vi "Autonomous Independent.vi"() -> ()   [LabVIEW 2011]
doc: "This VI is called when autonomous begins, and will automatically be terminated when autonomous ends. You can carry out timed or sensor driven robot movement independently without needing to return to the caller."
uses:
  <vilib>/addons/Kinect/Skeleton Vertex Index.ctl
  Robot Global Data.vi
  <vilib>/addons/control/pid/pid.llb/PID (DBL).vi
  <vilib>/addons/control/pid/NI_PID_pid.lvlib
panel:
  out "z 2":sgl
  out "y 2":sgl
  out "x 2":sgl
  out "z":sgl
  out "y":sgl
  out "x":sgl
  in  "PID gains":T1={"proportional gain (Kc)"=0.02, "integral time (Ti, min)"=0.0, "derivative time (Td, min)"=0.0}
  in  "setpoint":dbl=3000.0 format="%.2f"
  in  "PID gains 2":T1={"proportional gain (Kc)"=0.02, "integral time (Ti, min)"=0.0, "derivative time (Td, min)"=0.0}
  in  "setpoint 2":dbl=3300.0 format="%.2f"
  out "Left Distance 4":dbl
  out "Right Distance 4":dbl
  out "Right Distance 3":dbl
  out "Left Distance 3":dbl
  out "Left Distance 2":dbl
  out "Right Distance 2":dbl
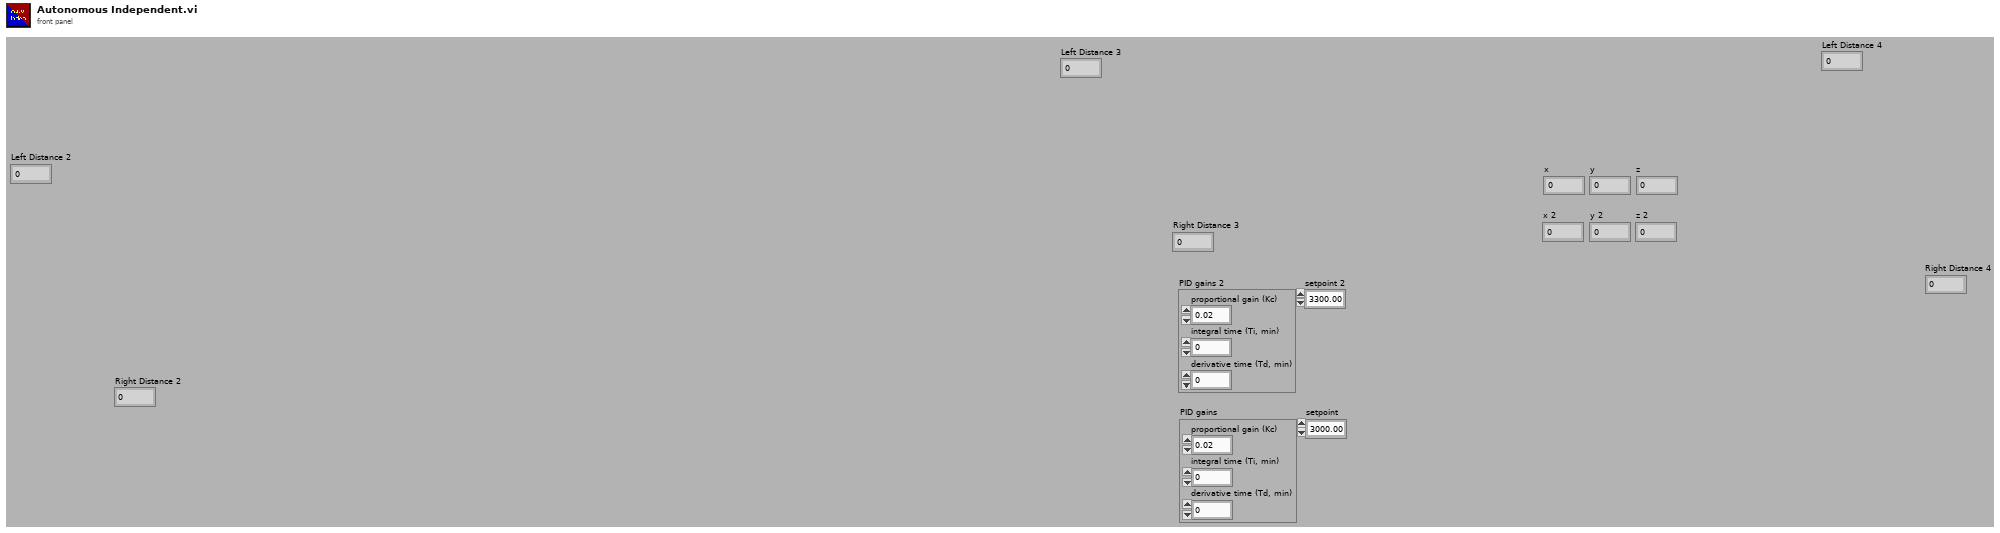
[diagram p1: front panel]
types:
  T1 = cluster{"proportional gain (Kc)":dbl, "integral time (Ti, min)":dbl, "derivative time (Td, min)":dbl}
  T2 = typedef "WPI_JoystickDevRef.ctl" = cluster{"Device":T3}
  T3 = typedef "WPI_JoystickDeviceEnum.ctl" = enum16{"USB 1", "USB 2", "USB 3", "USB 4", "Kinect 1", "Kinect 2"}
  T4 = cluster{"axis 1 (x)":dbl, "axis 2 (y)":dbl, "axis 3 (throttle)":dbl, "axis 4":dbl, "axis 5":dbl, "axis 6":dbl}
  T5 = typedef "Skeleton Vertex Index.ctl" = i32
  T6 = typedef "WPI_RobotDriveDevRef.ctl" = cluster{"DevStatus":errorcluster, "Motors[]":T7[], "Square Inputs":bool, "Max Output":dbl, "Isochronous":bool}
  T7 = typedef "WPI_MotorControlDeviceRef.ctl" = cluster{"DeviceStatus":errorcluster, "Type":enum16{"PWM", "CAN"}, "PWM":cluster{"Digital Module":T8, "PWM Channel":T9, "DeadBand":T10}, "CAN":cluster{"Device Number":u8, "Control Mode":T11, "Semaphore":T12, "Max Vout":dbl}, "Invert":bool, "TransformRef":T13, "InvTransformRef":T13}
  T8 = typedef "FPGA_TypedefDigitalModule.ctl" = enum16{"Digital Module 1", "Digital Module 2"}
  T9 = typedef "FPGA_DIOPWMChannel.ctl" = enum8{"PWM 1", "PWM 2", "PWM 3", "PWM 4", "PWM 5", "PWM 6", "PWM 7", "PWM 8", "PWM 9", "PWM 10", "Invalid"}
  T10 = typedef "WPI_PWMDeadband.ctl" = cluster{"Name":string, "maxPositivePwm":i32, "minPositivePwm":i32, "centerPwm":i32, "maxNegativePwm":i32, "minNegativePwm":i32, "angularRange":u16}
  T11 = typedef "WPI_CANJaguar_ControlMode.ctl" = enum8{"Percent VBus", "Current", "Speed", "Position", "Voltage"}
  T12 = typedef "Semaphore RefNum" = refnum<k1>
  T13 = typedef "WPI_PWMTransform_ConPane.ctl" = refnum<vi>
  T14 = typedef "WPI_EncoderDevRef.ctl" = cluster{"DevStatus":errorcluster, "EncoderIndex":T15, "CounterIndex":T16, "DistancePerCount":dbl, "Decoding Type":T17}
  T15 = typedef "FPGA_EncoderIdx.ctl" = enum8{"Enc 0", "Enc 1", "Enc 2", "Enc 3", "Invalid"}
  T16 = typedef "FPGA_CounterCtrSystemIndex.ctl" = enum8{"Ctr 0", "Ctr 1", "Ctr 2", "Ctr 3", "Ctr 4", "Ctr 5", "Ctr 6", "Ctr 7", "Invalid"}
  T17 = typedef "WPI_EncoderType.ctl" = enum16{"1x", "2x", "4x"}
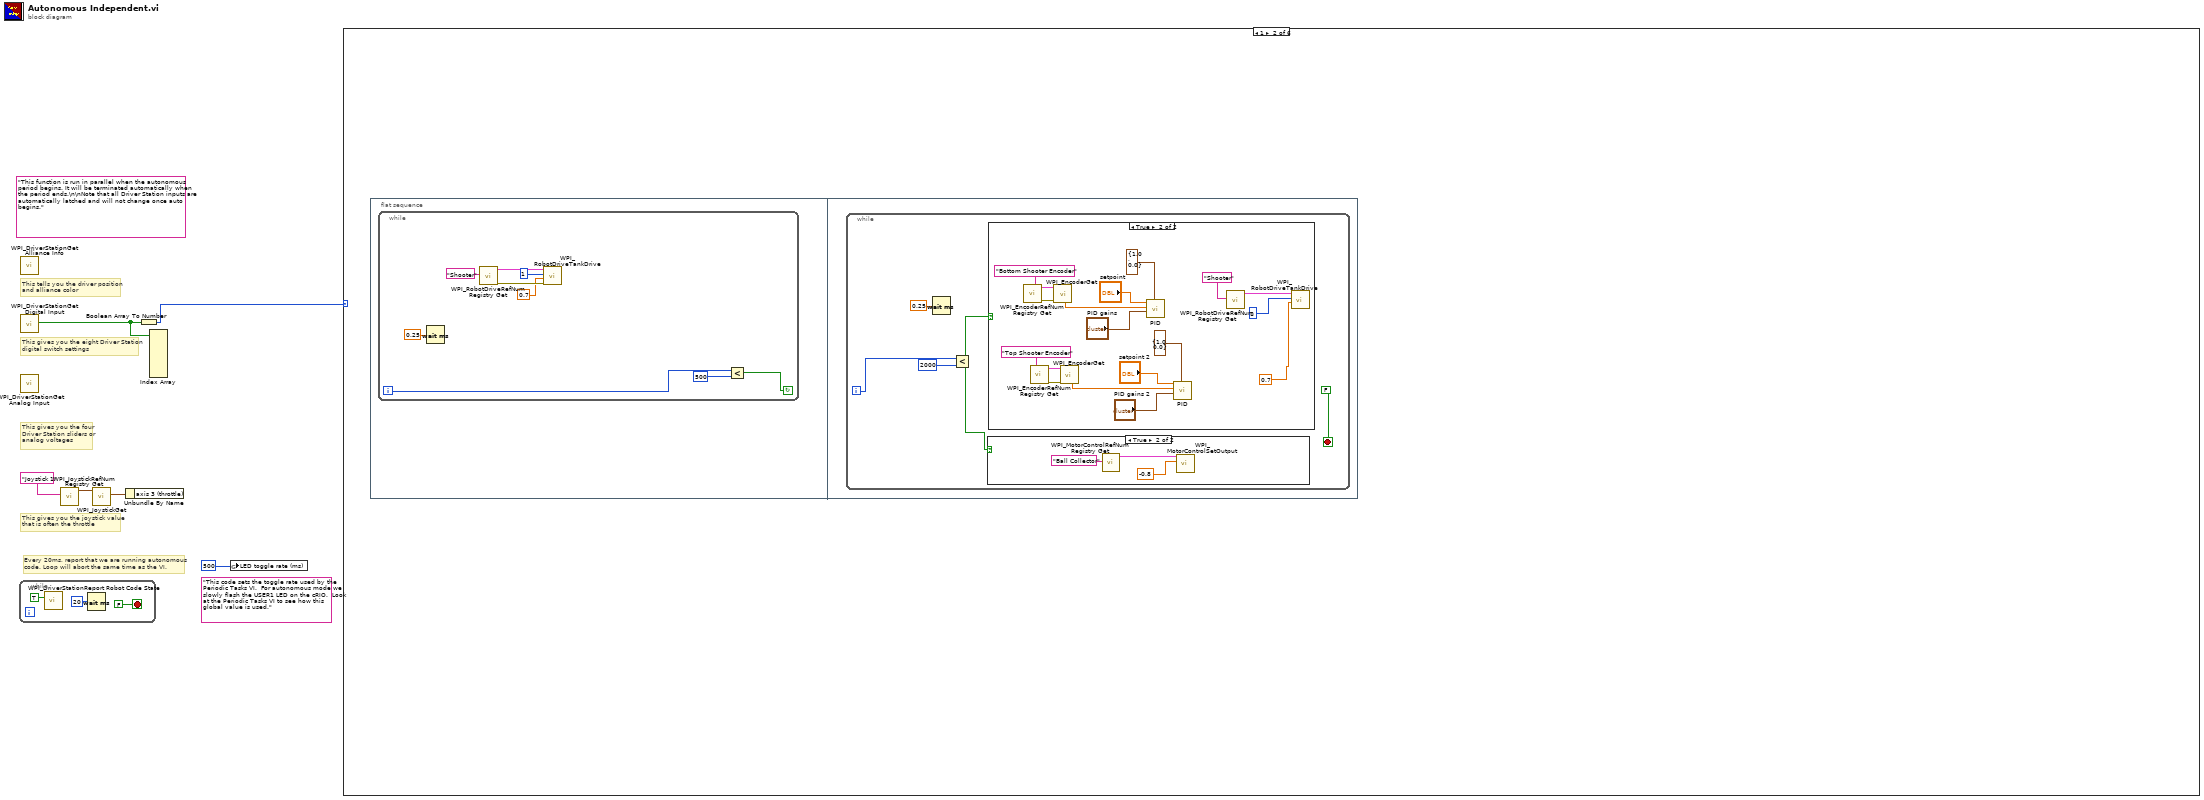
[diagram p0: block diagram]
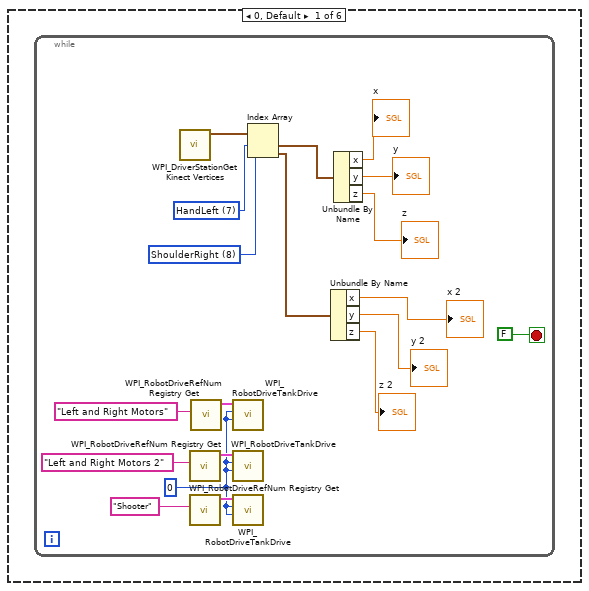
[diagram p2: hidden frame]
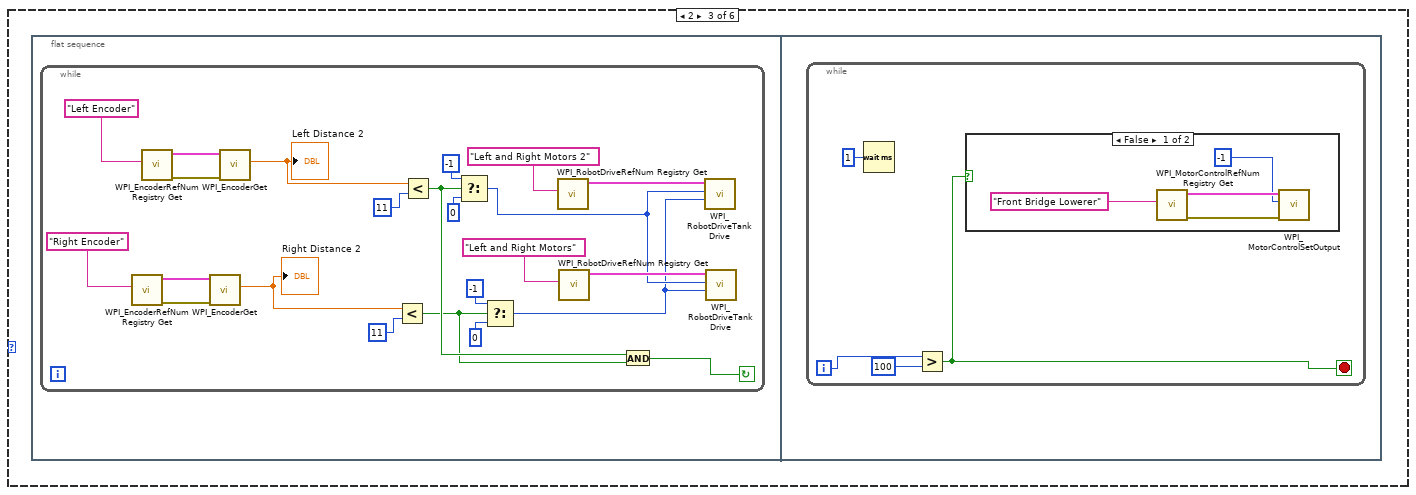
[diagram p5: hidden frame]
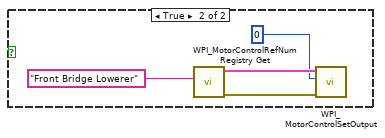
[diagram p6: hidden frame]
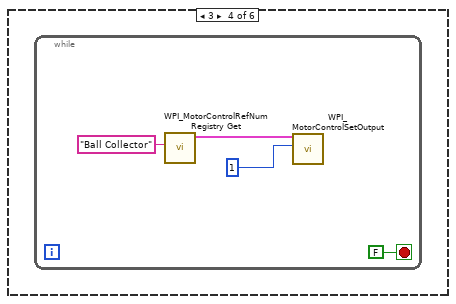
[diagram p7: hidden frame]
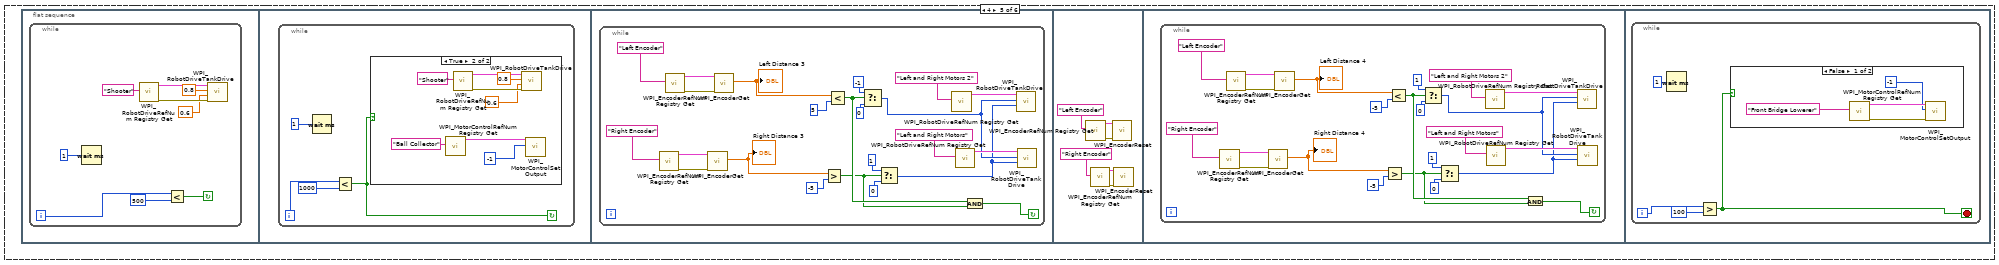
[diagram p8: hidden frame]
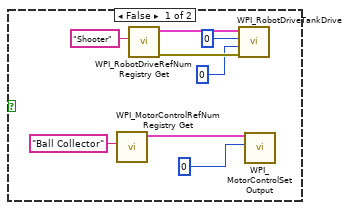
[diagram p9: hidden frame]
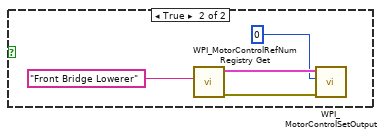
[diagram p10: hidden frame]
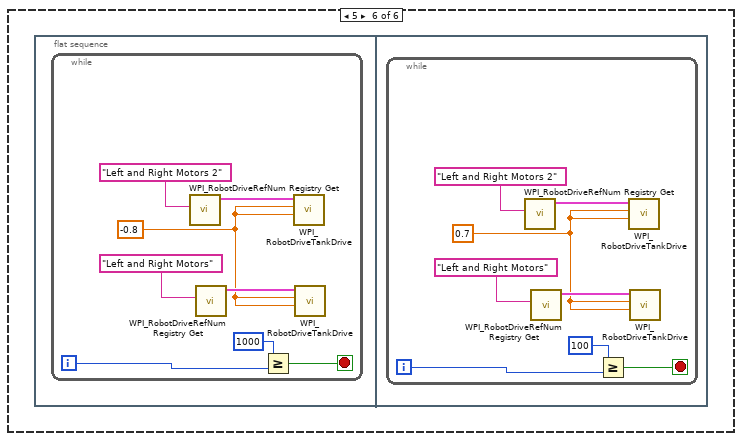
[diagram p11: hidden frame]
diagram:
  (unwired) "This code sets the toggle rate used by the Periodic Tasks VI.  For autonomous mode we slowly flash the USER1 LED on the cRIO.  Look at the Periodic Tasks VI to see how this global value is used."
  (unwired) "This function is run in parallel when the autonomous period begins. It will be terminated automatically when the period ends.\n\nNote that all Driver Station inputs are automatically latched and will not change once auto begins."
  # "Every 20ms, report that we are running autonomous\ncode. Loop will abort the same time as the VI."
  # "This gives you the joystick value\nthat is often the throttle"
  # "This tells you the driver position\nand alliance color"
  # "This gives you the eight Driver Station\ndigital switch settings"
  # "This gives you the four\nDriver Station sliders or\nanalog voltages"
  n1 = while {
    stop <- FALSE stop-if-true
    n2 = call <vilib>:"WPI_DriverStationReport Robot Code State.vi"("Autonomous"=TRUE) -> ()  [unwired: 10 in, 1 out]
    n3 = Wait (ms)(milliseconds to wait=u32 20) -> ()  [unwired: 1 out]
  }
  n4 = call <vilib>:"WPI_DriverStationGet Alliance Info.vi"() -> ()  [unwired: 12 out]
  n5 = call <vilib>:"WPI_DriverStationGet Digital Input.vi"() -> ("Driver Station Digital Input (1-8)"=w2:bool[])  [unwired: 11 out]
  n6 = call <vilib>:"WPI_DriverStationGet Analog Input.vi"() -> ()  [unwired: 12 out]
  n7 = call <vilib>:"WPI_JoystickRefNum Registry Get.vi"("refnum name"="Joystick 1") -> ("JoystickDevRef"=w4:T2)  [unwired: 1 in, 9 out]
  n8 = call <vilib>:"WPI_JoystickGet.vi"("JoystickDevRef"=w4) -> ("Axes"=w5:T4)  [unwired: 1 in, 5 out]
  n9 = Unbundle By Name(w5) -> ()  [unwired: 1 out]
  n10 = Boolean Array To Number(Boolean array=w2) -> (number=w1:u32)
  n11 = Index Array(array=w2) -> ()  [unwired: 8 in, 8 out]
  n12 = global write "Robot Global Data.vi" "LED toggle rate (ms)"(u32 500 ("LED ms toggle rate")) -> ()
  n13 = case shown="1" w1 {
    frame 0, Default {
      n14 = while {
        stop <- FALSE stop-if-true
        w13 = 0
        w20 = T5 8 items=["HipCenter", "Spine", "ShoulderCenter", "Head", "ShoulderLeft", "ElbowLeft", "WristLeft", "HandLeft", "ShoulderRight", "ElbowRight", "WristRight", "HandRight", "HipLeft", "KneeLeft", "AnkleLeft", "FootLeft", "HipRight", "KneeRight", "AnkleRight", "FootRight"] ("Skeleton Joints")
        w27 = T5 7 items=["HipCenter", "Spine", "ShoulderCenter", "Head", "ShoulderLeft", "ElbowLeft", "WristLeft", "HandLeft", "ShoulderRight", "ElbowRight", "WristRight", "HandRight", "HipLeft", "KneeLeft", "AnkleLeft", "FootLeft", "HipRight", "KneeRight", "AnkleRight", "FootRight"] ("Skeleton Joints")
        n15 = call <vilib>:"WPI_DriverStationGet Kinect Vertices.vi"() -> ("Skeleton Vertices"=w28:cluster{"x":sgl, "y":sgl, "z":sgl}[])  [unwired: 10 in, 1 out]
        n16 = call <vilib>:"WPI_RobotDriveRefNum Registry Get.vi"("refnum name"="Left and Right Motors 2") -> ("RobotDriveDevRef"=w15:T6)  [unwired: 9 in, 1 out]
        n17 = call <vilib>:"WPI_RobotDriveRefNum Registry Get.vi"("refnum name"="Shooter") -> ("RobotDriveDevRef"=w14:T6)  [unwired: 9 in, 1 out]
        n18 = call <vilib>:"WPI_RobotDriveRefNum Registry Get.vi"("refnum name"="Left and Right Motors") -> ("RobotDriveDevRef"=w16:T6)  [unwired: 9 in, 1 out]
        n19 = call <vilib>:"WPI_RobotDriveTankDrive.vi"("Right axis value"=w13, "Left axis value"=w13, "RobotDriveDevRef"=w16) -> ()  [unwired: 7 in, 2 out]
        n20 = call <vilib>:"WPI_RobotDriveTankDrive.vi"("Right axis value"=w13, "Left axis value"=w13, "RobotDriveDevRef"=w15) -> ()  [unwired: 7 in, 2 out]
        n21 = call <vilib>:"WPI_RobotDriveTankDrive.vi"("Right axis value"=w13, "Left axis value"=w13, "RobotDriveDevRef"=w14) -> ()  [unwired: 7 in, 2 out]
        n22 = Index Array(array=w28, index #1=w27, index #2=w20) -> (element #1=w26:cluster{"x":sgl, "y":sgl, "z":sgl}, element #2=w21:cluster{"x":sgl, "y":sgl, "z":sgl})
        n23 = Unbundle By Name(w21) -> ("x"=→"x 2":sgl, "y"=→"y 2":sgl, "z"=→"z 2":sgl)
        n24 = Unbundle By Name(w26) -> ("x"=→"x":sgl, "y"=→"y":sgl, "z"=→"z":sgl)
      }
    }
    frame 1 {
      n25 = flat-sequence {
        frame #0 {
          n26 = while {
            i -> [w36]
            stop <- w35 continue-if-true
            n27 = Wait (ms)(milliseconds to wait=0.25) -> ()  [unwired: 1 out]
            n28 = call <vilib>:"WPI_RobotDriveRefNum Registry Get.vi"("refnum name"="Shooter") -> ("error out"=w33:errorcluster, "RobotDriveDevRef"=w32:T6)  [unwired: 9 in]
            n29 = call <vilib>:"WPI_RobotDriveTankDrive.vi"("error in (no error)"=w33, "Right axis value"=0.7, "Left axis value"=1, "RobotDriveDevRef"=w32) -> ()  [unwired: 6 in, 2 out]
            n30 = Less?(x=w36, y=500) -> (x < y?=w35:bool)
          }
        }
        frame #1 {
          n31 = while {
            i -> [w40]
            stop <- FALSE stop-if-true
            n32 = Wait (ms)(milliseconds to wait=0.25) -> ()  [unwired: 1 out]
            n33 = Less?(x=w40, y=2000) -> (x < y?=w38:bool)
            n34 = case shown="True" w38 {
              frame False {
              }
              frame True {
                n35 = call <vilib>:"WPI_MotorControlRefNum Registry Get.vi"("refnum name"="Ball Collector") -> ("MotorControlDevRef"=w44:T7)  [unwired: 9 in, 1 out]
                n36 = call <vilib>:"WPI_MotorControlSetOutput.vi"("Output"=-0.8, "MotorControlDevRef"=w44) -> ()  [unwired: 8 in, 2 out]
              }
            }
            n37 = case shown="True" w38 {
              frame False {
              }
              frame True {
                n38 = call <vilib>:"WPI_EncoderRefNum Registry Get.vi"("refnum name"="Bottom Shooter Encoder") -> ("error out"=w51:errorcluster, "EncoderDevRef"=w52:T14)  [unwired: 9 in]
                n39 = call <vilib>:"WPI_EncoderRefNum Registry Get.vi"("refnum name"="Top Shooter Encoder") -> ("error out"=w54:errorcluster, "EncoderDevRef"=w55:T14)  [unwired: 9 in]
                n40 = call <vilib>:"WPI_EncoderGet.vi"("error in (no error)"=w51, "EncoderDevRef"=w52) -> ("Rate"=w49:dbl)  [unwired: 4 in, 5 out]
                n41 = call <vilib>:"WPI_EncoderGet.vi"("error in (no error)"=w54, "EncoderDevRef"=w55) -> ("Rate"=w48:dbl)  [unwired: 4 in, 5 out]
                n42 = call-poly <vilib>:"PID.vi"("output range"=cluster{"output high":dbl, "output low":dbl} {"output high"=1.0, "output low"=0.0}, "PID gains"="PID gains", "process variable"=w49, "setpoint"="setpoint") -> ()  [unwired: 6 in, 2 out]
                n43 = call-poly <vilib>:"PID.vi"("output range"=cluster{"output high":dbl, "output low":dbl} {"output high"=1.0, "output low"=0.0}, "PID gains"="PID gains 2", "process variable"=w48, "setpoint"="setpoint 2") -> ()  [unwired: 6 in, 2 out]
                n44 = call <vilib>:"WPI_RobotDriveRefNum Registry Get.vi"("refnum name"="Shooter") -> ("RobotDriveDevRef"=w63:T6)  [unwired: 1 in, 9 out]
                n45 = call <vilib>:"WPI_RobotDriveTankDrive.vi"("Right axis value"=0.7, "Left axis value"=1, "RobotDriveDevRef"=w63) -> ()  [unwired: 7 in, 2 out]
              }
            }
          }
        }
      }
    }
    frame 2 {
      n46 = flat-sequence {
        frame #0 {
          n47 = while {
            stop <- w64 continue-if-true
            n48 = call <vilib>:"WPI_EncoderRefNum Registry Get.vi"("refnum name"="Right Encoder") -> ("error out"=w82:errorcluster, "EncoderDevRef"=w83:T14)  [unwired: 9 in]
            n49 = call <vilib>:"WPI_EncoderRefNum Registry Get.vi"("refnum name"="Left Encoder") -> ("error out"=w85:errorcluster, "EncoderDevRef"=w84:T14)  [unwired: 9 in]
            n50 = call <vilib>:"WPI_EncoderGet.vi"("error in (no error)"=w82, "EncoderDevRef"=w83) -> ("Distance"=w69:dbl)  [unwired: 4 in, 5 out]
            "Right Distance 2" <- w69
            n51 = call <vilib>:"WPI_EncoderGet.vi"("error in (no error)"=w85, "EncoderDevRef"=w84) -> ("Distance"=w75:dbl)  [unwired: 4 in, 5 out]
            "Left Distance 2" <- w75
            n52 = Less?(x=w69, y=11) -> (x < y?=w65:bool)
            n53 = Less?(x=w75, y=11) -> (x < y?=w66:bool)
            n54 = Select(t=-1, s=w66, f=0) -> (s? t:f=w72:i32)
            n55 = Select(t=-1, s=w65, f=0) -> (s? t:f=w67:i32)
            n56 = call <vilib>:"WPI_RobotDriveRefNum Registry Get.vi"("refnum name"="Left and Right Motors 2") -> ("RobotDriveDevRef"=w80:T6)  [unwired: 1 in, 9 out]
            n57 = call <vilib>:"WPI_RobotDriveRefNum Registry Get.vi"("refnum name"="Left and Right Motors") -> ("RobotDriveDevRef"=w78:T6)  [unwired: 1 in, 9 out]
            n58 = And(x=w66, y=w65) -> (x .and. y?=w64:bool)
            n59 = call <vilib>:"WPI_RobotDriveTankDrive.vi"("Right axis value"=w67, "Left axis value"=w72, "RobotDriveDevRef"=w80) -> ()  [unwired: 7 in, 2 out]
            n60 = call <vilib>:"WPI_RobotDriveTankDrive.vi"("Right axis value"=w67, "Left axis value"=w72, "RobotDriveDevRef"=w78) -> ()  [unwired: 7 in, 2 out]
          }
        }
        frame #1 {
          n61 = while {
            i -> [w90]
            stop <- w88 stop-if-true
            n62 = Wait (ms)(milliseconds to wait=u32 1) -> ()  [unwired: 1 out]
            n63 = Greater?(x=w90, y=100) -> (0:w88:bool)
            n64 = case shown="False" w88 {
              frame False {
                n65 = call <vilib>:"WPI_MotorControlRefNum Registry Get.vi"("refnum name"="Front Bridge Lowerer") -> ("error out"=w93:errorcluster, "MotorControlDevRef"=w94:T7)  [unwired: 9 in]
                n66 = call <vilib>:"WPI_MotorControlSetOutput.vi"("error in (no error)"=w93, "Output"=-1, "MotorControlDevRef"=w94) -> ()  [unwired: 7 in, 2 out]
              }
              frame True {
                n67 = call <vilib>:"WPI_MotorControlRefNum Registry Get.vi"("refnum name"="Front Bridge Lowerer") -> ("error out"=w97:errorcluster, "MotorControlDevRef"=w98:T7)  [unwired: 9 in]
                n68 = call <vilib>:"WPI_MotorControlSetOutput.vi"("error in (no error)"=w97, "Output"=0, "MotorControlDevRef"=w98) -> ()  [unwired: 7 in, 2 out]
              }
            }
          }
        }
      }
    }
    frame 3 {
      n69 = while {
        stop <- FALSE stop-if-true
        n70 = call <vilib>:"WPI_MotorControlRefNum Registry Get.vi"("refnum name"="Ball Collector") -> ("MotorControlDevRef"=w101:T7)  [unwired: 9 in, 1 out]
        n71 = call <vilib>:"WPI_MotorControlSetOutput.vi"("Output"=1, "MotorControlDevRef"=w101) -> ()  [unwired: 8 in, 2 out]
      }
    }
    frame 4 {
      n72 = flat-sequence {
        frame #0 {
          n73 = while {
            i -> [w110]
            stop <- w109 continue-if-true
            n74 = Wait (ms)(milliseconds to wait=1) -> ()  [unwired: 1 out]
            n75 = call <vilib>:"WPI_RobotDriveRefNum Registry Get.vi"("refnum name"="Shooter") -> ("error out"=w107:errorcluster, "RobotDriveDevRef"=w106:T6)  [unwired: 9 in]
            n76 = Less?(x=w110, y=500) -> (x < y?=w109:bool)
            n77 = call <vilib>:"WPI_RobotDriveTankDrive.vi"("error in (no error)"=w107, "Right axis value"=0.6, "Left axis value"=0.8, "RobotDriveDevRef"=w106) -> ()  [unwired: 6 in, 2 out]
          }
        }
        frame #1 {
          n78 = while {
            i -> [w114]
            stop <- w112 continue-if-true
            n79 = Wait (ms)(milliseconds to wait=1) -> ()  [unwired: 1 out]
            n80 = Less?(x=w114, y=1000) -> (x < y?=w112:bool)
            n81 = case shown="True" w112 {
              frame False {
                n82 = call <vilib>:"WPI_MotorControlRefNum Registry Get.vi"("refnum name"="Ball Collector") -> ("MotorControlDevRef"=w117:T7)  [unwired: 9 in, 1 out]
                n83 = call <vilib>:"WPI_RobotDriveRefNum Registry Get.vi"("refnum name"="Shooter") -> ("error out"=w122:errorcluster, "RobotDriveDevRef"=w121:T6)  [unwired: 9 in]
                n84 = call <vilib>:"WPI_RobotDriveTankDrive.vi"("error in (no error)"=w122, "Right axis value"=0, "Left axis value"=0, "RobotDriveDevRef"=w121) -> ()  [unwired: 6 in, 2 out]
                n85 = call <vilib>:"WPI_MotorControlSetOutput.vi"("Output"=0, "MotorControlDevRef"=w117) -> ()  [unwired: 8 in, 2 out]
              }
              frame True {
                n86 = call <vilib>:"WPI_MotorControlRefNum Registry Get.vi"("refnum name"="Ball Collector") -> ("MotorControlDevRef"=w125:T7)  [unwired: 9 in, 1 out]
                n87 = call <vilib>:"WPI_RobotDriveRefNum Registry Get.vi"("refnum name"="Shooter") -> ("error out"=w130:errorcluster, "RobotDriveDevRef"=w129:T6)  [unwired: 9 in]
                n88 = call <vilib>:"WPI_RobotDriveTankDrive.vi"("error in (no error)"=w130, "Right axis value"=0.6, "Left axis value"=0.8, "RobotDriveDevRef"=w129) -> ()  [unwired: 6 in, 2 out]
                n89 = call <vilib>:"WPI_MotorControlSetOutput.vi"("Output"=-1, "MotorControlDevRef"=w125) -> ()  [unwired: 8 in, 2 out]
              }
            }
          }
        }
        frame #2 {
          n90 = while {
            stop <- w133 continue-if-true
            n91 = call <vilib>:"WPI_EncoderRefNum Registry Get.vi"("refnum name"="Right Encoder") -> ("error out"=w150:errorcluster, "EncoderDevRef"=w151:T14)  [unwired: 9 in]
            n92 = call <vilib>:"WPI_EncoderRefNum Registry Get.vi"("refnum name"="Left Encoder") -> ("error out"=w153:errorcluster, "EncoderDevRef"=w152:T14)  [unwired: 9 in]
            n93 = call <vilib>:"WPI_EncoderGet.vi"("error in (no error)"=w150, "EncoderDevRef"=w151) -> ("Distance"=w138:dbl)  [unwired: 4 in, 5 out]
            "Right Distance 3" <- w138
            n94 = call <vilib>:"WPI_EncoderGet.vi"("error in (no error)"=w153, "EncoderDevRef"=w152) -> ("Distance"=w144:dbl)  [unwired: 4 in, 5 out]
            "Left Distance 3" <- w144
            n95 = Greater?(x=w138, y=-5) -> (0:w134:bool)
            n96 = Less?(x=w144, y=5) -> (x < y?=w135:bool)
            n97 = Select(t=-1, s=w135, f=0) -> (s? t:f=w141:i32)
            n98 = Select(t=1, s=w134, f=0) -> (s? t:f=w136:i32)
            n99 = call <vilib>:"WPI_RobotDriveRefNum Registry Get.vi"("refnum name"="Left and Right Motors 2") -> ("RobotDriveDevRef"=w148:T6)  [unwired: 1 in, 9 out]
            n100 = call <vilib>:"WPI_RobotDriveRefNum Registry Get.vi"("refnum name"="Left and Right Motors") -> ("RobotDriveDevRef"=w146:T6)  [unwired: 1 in, 9 out]
            n101 = And(x=w135, y=w134) -> (x .and. y?=w133:bool)
            n102 = call <vilib>:"WPI_RobotDriveTankDrive.vi"("Right axis value"=w136, "Left axis value"=w141, "RobotDriveDevRef"=w148) -> ()  [unwired: 7 in, 2 out]
            n103 = call <vilib>:"WPI_RobotDriveTankDrive.vi"("Right axis value"=w136, "Left axis value"=w141, "RobotDriveDevRef"=w146) -> ()  [unwired: 7 in, 2 out]
          }
        }
        frame #3 {
          n104 = call <vilib>:"WPI_EncoderRefNum Registry Get.vi"("refnum name"="Left Encoder") -> ("error out"=w158:errorcluster, "EncoderDevRef"=w157:T14)  [unwired: 9 in]
          n105 = call <vilib>:"WPI_EncoderRefNum Registry Get.vi"("refnum name"="Right Encoder") -> ("error out"=w155:errorcluster, "EncoderDevRef"=w156:T14)  [unwired: 9 in]
          n106 = call <vilib>:"WPI_EncoderReset.vi"("error in (no error)"=w158, "EncoderDevRef"=w157) -> ()  [unwired: 8 in, 2 out]
          n107 = call <vilib>:"WPI_EncoderReset.vi"("error in (no error)"=w155, "EncoderDevRef"=w156) -> ()  [unwired: 8 in, 2 out]
        }
        frame #4 {
          n108 = while {
            stop <- w162 continue-if-true
            n109 = call <vilib>:"WPI_EncoderRefNum Registry Get.vi"("refnum name"="Right Encoder") -> ("error out"=w179:errorcluster, "EncoderDevRef"=w180:T14)  [unwired: 9 in]
            n110 = call <vilib>:"WPI_EncoderRefNum Registry Get.vi"("refnum name"="Left Encoder") -> ("error out"=w182:errorcluster, "EncoderDevRef"=w181:T14)  [unwired: 9 in]
            n111 = call <vilib>:"WPI_EncoderGet.vi"("error in (no error)"=w179, "EncoderDevRef"=w180) -> ("Distance"=w167:dbl)  [unwired: 4 in, 5 out]
            "Right Distance 4" <- w167
            n112 = call <vilib>:"WPI_EncoderGet.vi"("error in (no error)"=w182, "EncoderDevRef"=w181) -> ("Distance"=w173:dbl)  [unwired: 4 in, 5 out]
            "Left Distance 4" <- w173
            n113 = Greater?(x=w167, y=-5) -> (0:w163:bool)
            n114 = Less?(x=w173, y=-5) -> (x < y?=w164:bool)
            n115 = Select(t=1, s=w164, f=0) -> (s? t:f=w170:i32)
            n116 = Select(t=1, s=w163, f=0) -> (s? t:f=w165:i32)
            n117 = call <vilib>:"WPI_RobotDriveRefNum Registry Get.vi"("refnum name"="Left and Right Motors 2") -> ("RobotDriveDevRef"=w177:T6)  [unwired: 1 in, 9 out]
            n118 = call <vilib>:"WPI_RobotDriveRefNum Registry Get.vi"("refnum name"="Left and Right Motors") -> ("RobotDriveDevRef"=w175:T6)  [unwired: 1 in, 9 out]
            n119 = And(x=w164, y=w163) -> (x .and. y?=w162:bool)
            n120 = call <vilib>:"WPI_RobotDriveTankDrive.vi"("Right axis value"=w165, "Left axis value"=w170, "RobotDriveDevRef"=w177) -> ()  [unwired: 7 in, 2 out]
            n121 = call <vilib>:"WPI_RobotDriveTankDrive.vi"("Right axis value"=w165, "Left axis value"=w170, "RobotDriveDevRef"=w175) -> ()  [unwired: 7 in, 2 out]
          }
        }
        frame #5 {
          n122 = while {
            i -> [w187]
            stop <- w185 stop-if-true
            n123 = Wait (ms)(milliseconds to wait=u32 1) -> ()  [unwired: 1 out]
            n124 = Greater?(x=w187, y=100) -> (0:w185:bool)
            n125 = case shown="False" w185 {
              frame False {
                n126 = call <vilib>:"WPI_MotorControlRefNum Registry Get.vi"("refnum name"="Front Bridge Lowerer") -> ("error out"=w190:errorcluster, "MotorControlDevRef"=w191:T7)  [unwired: 9 in]
                n127 = call <vilib>:"WPI_MotorControlSetOutput.vi"("error in (no error)"=w190, "Output"=-1, "MotorControlDevRef"=w191) -> ()  [unwired: 7 in, 2 out]
              }
              frame True {
                n128 = call <vilib>:"WPI_MotorControlRefNum Registry Get.vi"("refnum name"="Front Bridge Lowerer") -> ("error out"=w194:errorcluster, "MotorControlDevRef"=w195:T7)  [unwired: 9 in]
                n129 = call <vilib>:"WPI_MotorControlSetOutput.vi"("error in (no error)"=w194, "Output"=0, "MotorControlDevRef"=w195) -> ()  [unwired: 7 in, 2 out]
              }
            }
          }
        }
      }
    }
    frame 5 {
      n130 = flat-sequence {
        frame #0 {
          n131 = while {
            i -> [w197]
            stop <- w196 stop-if-true
            w199 = -0.8
            n132 = call <vilib>:"WPI_RobotDriveRefNum Registry Get.vi"("refnum name"="Left and Right Motors 2") -> ("RobotDriveDevRef"=w203:T6)  [unwired: 1 in, 9 out]
            n133 = call <vilib>:"WPI_RobotDriveRefNum Registry Get.vi"("refnum name"="Left and Right Motors") -> ("RobotDriveDevRef"=w201:T6)  [unwired: 1 in, 9 out]
            n134 = Greater Or Equal?(x=1000, y=w197) -> (x >= y?=w196:bool)
            n135 = call <vilib>:"WPI_RobotDriveTankDrive.vi"("Right axis value"=w199, "Left axis value"=w199, "RobotDriveDevRef"=w203) -> ()  [unwired: 7 in, 2 out]
            n136 = call <vilib>:"WPI_RobotDriveTankDrive.vi"("Right axis value"=w199, "Left axis value"=w199, "RobotDriveDevRef"=w201) -> ()  [unwired: 7 in, 2 out]
          }
        }
        frame #1 {
          n137 = while {
            i -> [w205]
            stop <- w204 stop-if-true
            w207 = 0.7
            n138 = call <vilib>:"WPI_RobotDriveRefNum Registry Get.vi"("refnum name"="Left and Right Motors 2") -> ("RobotDriveDevRef"=w211:T6)  [unwired: 1 in, 9 out]
            n139 = call <vilib>:"WPI_RobotDriveRefNum Registry Get.vi"("refnum name"="Left and Right Motors") -> ("RobotDriveDevRef"=w209:T6)  [unwired: 1 in, 9 out]
            n140 = Greater Or Equal?(x=100, y=w205) -> (x >= y?=w204:bool)
            n141 = call <vilib>:"WPI_RobotDriveTankDrive.vi"("Right axis value"=w207, "Left axis value"=w207, "RobotDriveDevRef"=w211) -> ()  [unwired: 7 in, 2 out]
            n142 = call <vilib>:"WPI_RobotDriveTankDrive.vi"("Right axis value"=w207, "Left axis value"=w207, "RobotDriveDevRef"=w209) -> ()  [unwired: 7 in, 2 out]
          }
        }
      }
    }
  }
